vi "Main.vi"() -> ()   [LabVIEW 2022 SP3]
doc: "This Continuous Measurement sample project is based on the Queued Message Handler template.\n\nThe Event Handling Loop generates messages based on user interface actions.\n\nThe Message Handling Loop processes messages generated by the Event Handling Loop, or by other messages. There are also Acquisition and Logging message handling loop subVIs, and a chart updating loop."
uses:
  controls/UI Data.ctl
  controls/UI State.ctl
  support/Message Queue/Enqueue Message (Single).vi
  GlobalVariable/GlobalLongueurOnde.vi
  GlobalVariable/GlobalSet0.vi
  GlobalVariable/GlobalDefaultFolderPath.vi
  <vilib>/Utility/error.llb/Error Cluster From Error Code.vi
  <vilib>/ErrorRing/Error Ring.xnode
  Acquisition/Acquisition.lvlib
  support/User Event - Stop/User Event - Stop.lvlib
  support/Message Queue/Message Queue.lvlib
panel:
  out "Pos Y":dbl
  out "Pos X":dbl
  out "?":dbl[][](graph)
  in  "Mise à 0":bool
  in  "Longueur d'onde du laser":dbl
  in  "Exit":bool
  out "Data":waveform(dbl)[](graph)
  out "Array":variant[](array[variant])
  out "Status":string
  out "Puissance Instantannée":dbl
  in  "Start":bool
  in  "Stop":bool
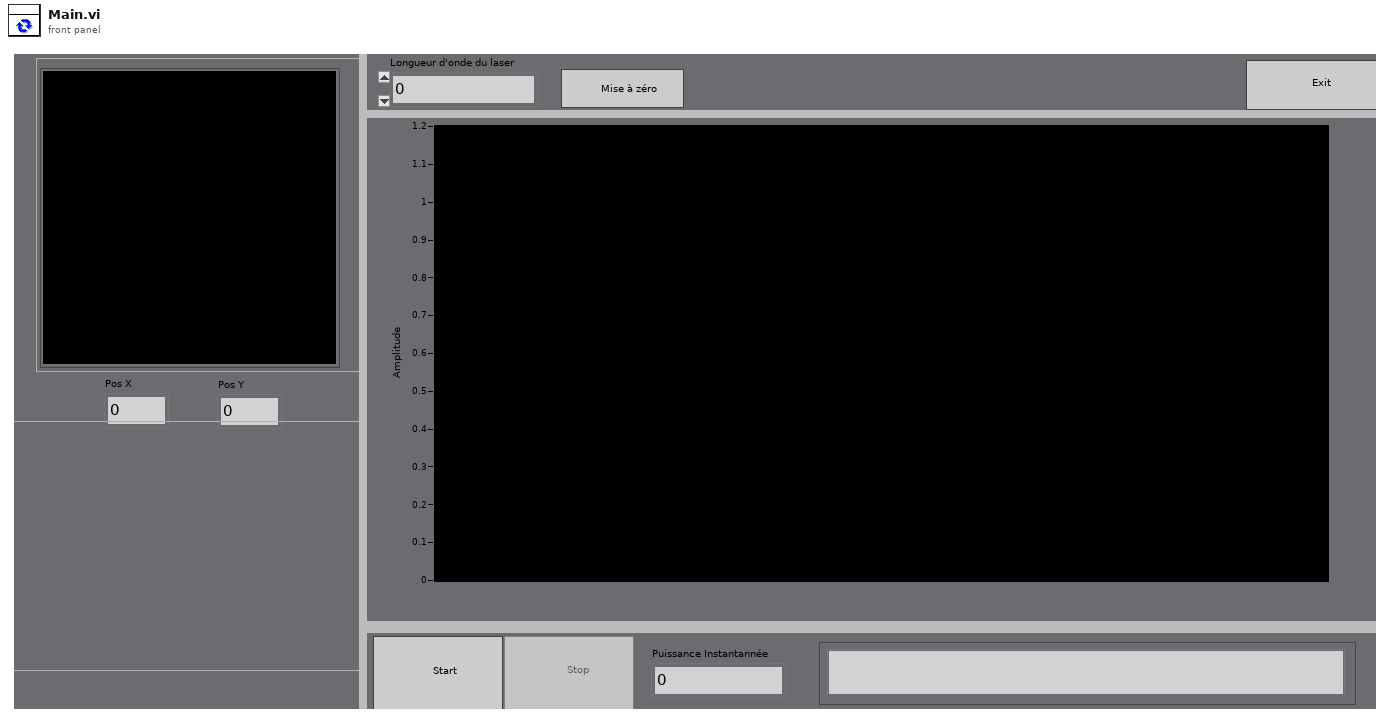
[diagram p1: front panel]
types:
  T1 = typedef "UI State.ctl" = enum16{"Idle", "Acquiring and Logging", "Waiting for Exit", "Waiting for Exit (Acq Stopped)", "Waiting for Exit (Log Stopped)", "Waiting for Stop", "Waiting for Stop (Acq Stopped)", "Waiting for Stop (Log Stopped)"}
  T2 = typedef "UI Data.ctl" = cluster{"Start Ref":refnum<vi>, "Stop Ref":refnum<vi>, "Settings Ref":refnum<vi>, "Exit Ref":refnum<vi>, "Status Ref":refnum<vi>, "Data Ref":refnum<vi>, "Longueur d'onde du laser":refnum<vi>, "Set 0 Ref":refnum<vi>}
  T3 = cluster{"UI":refnum<queue>, "Acquisition":refnum<queue>}
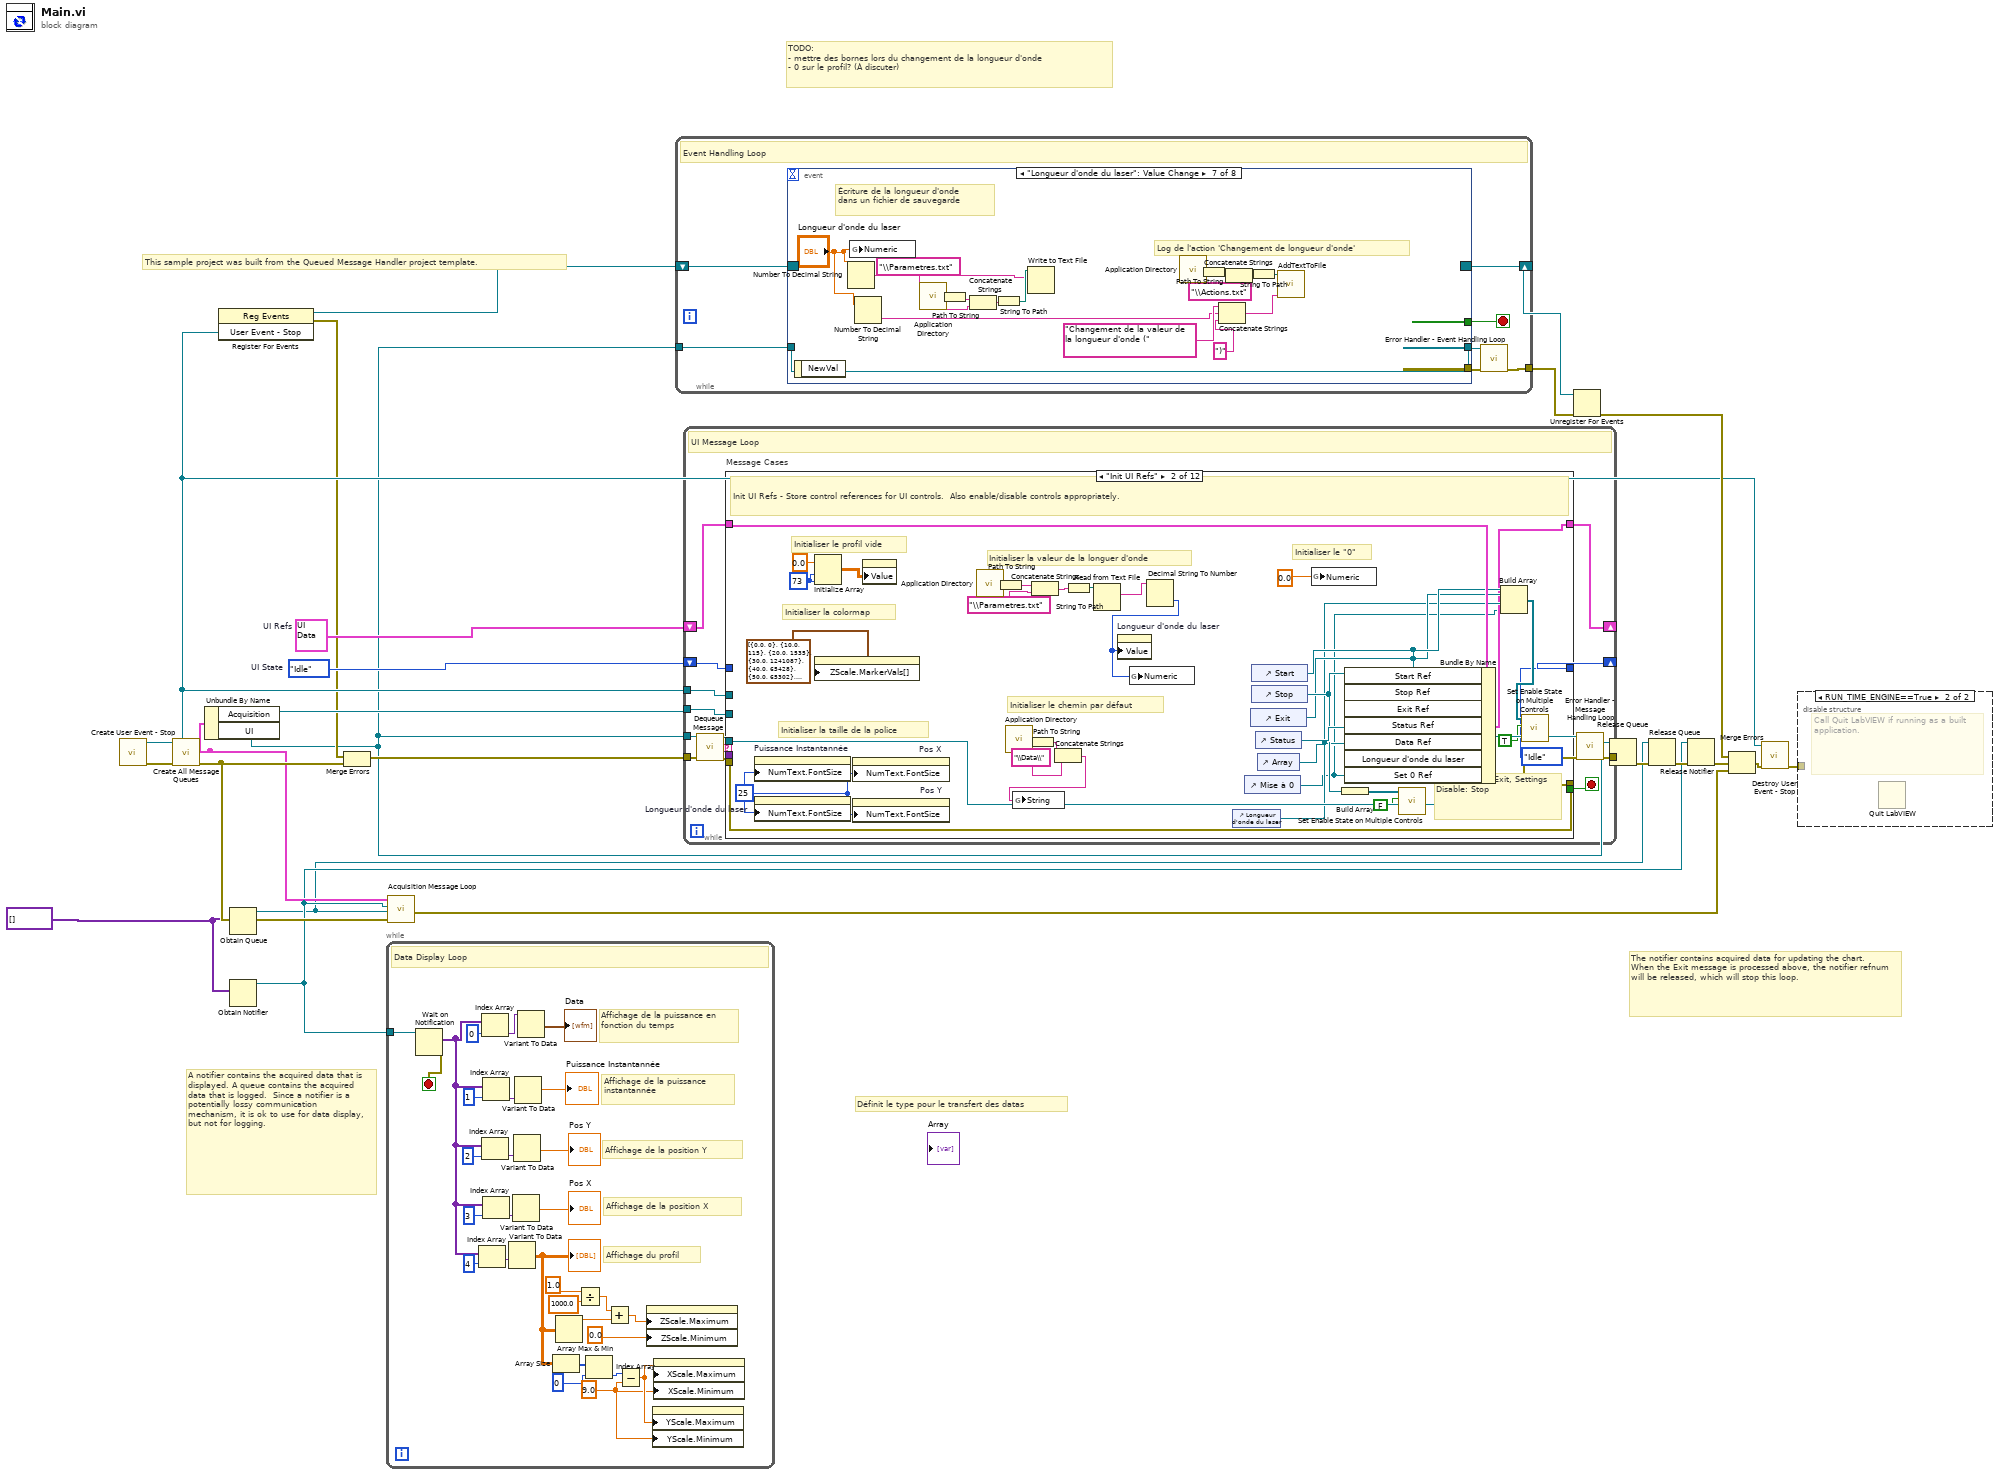
[diagram p0: block diagram]
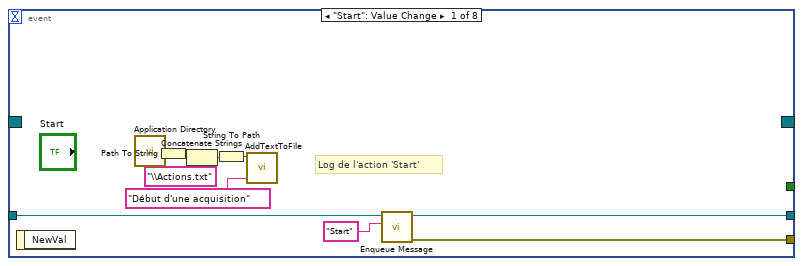
[diagram p3: hidden frame]
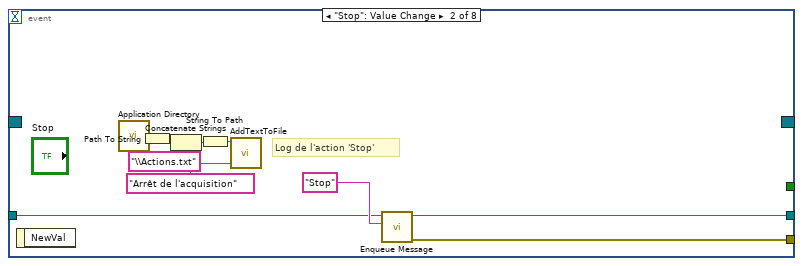
[diagram p4: hidden frame]
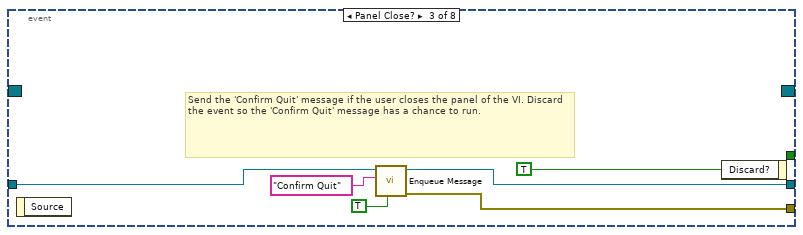
[diagram p5: hidden frame]
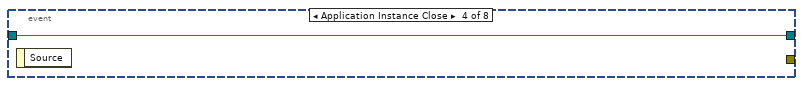
[diagram p6: hidden frame]
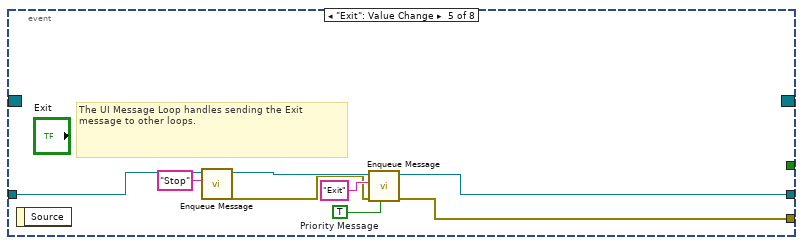
[diagram p7: hidden frame]
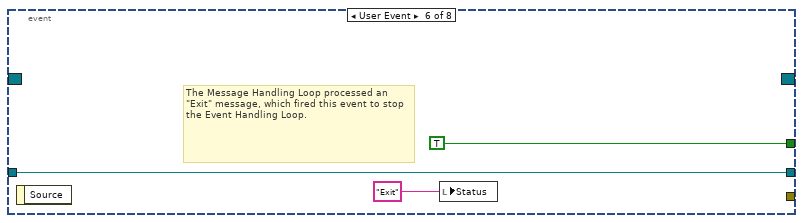
[diagram p8: hidden frame]
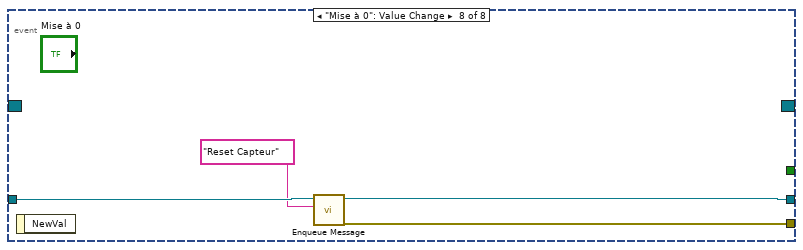
[diagram p9: hidden frame]
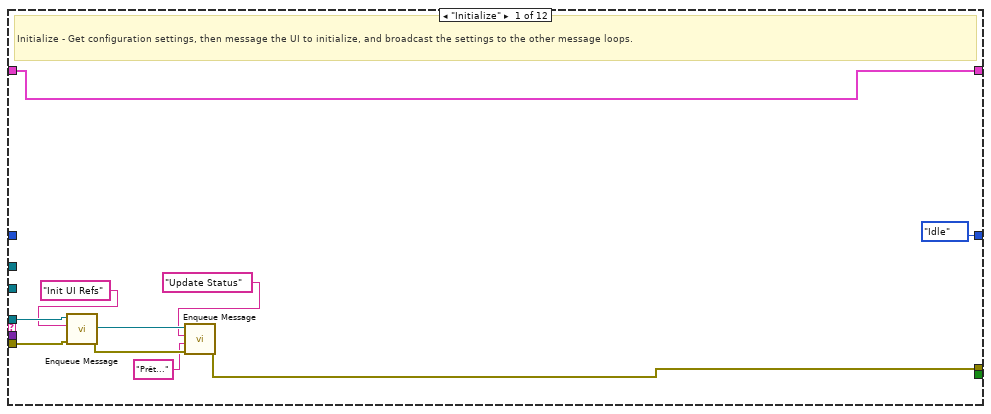
[diagram p10: hidden frame]
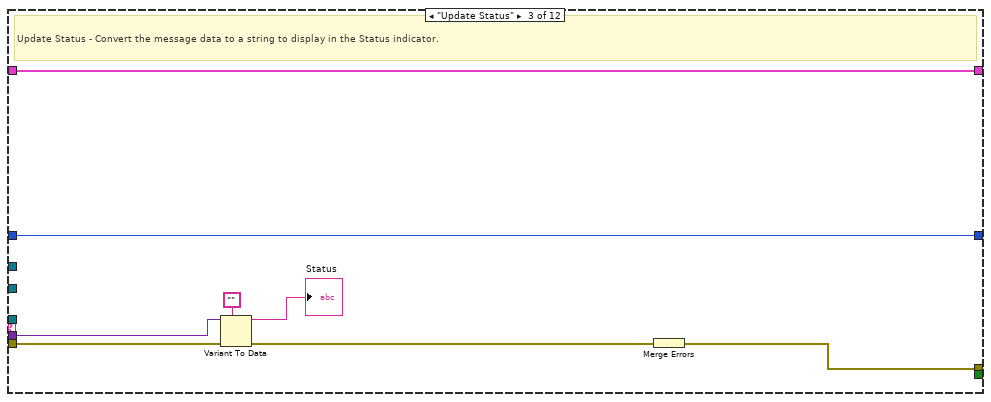
[diagram p11: hidden frame]
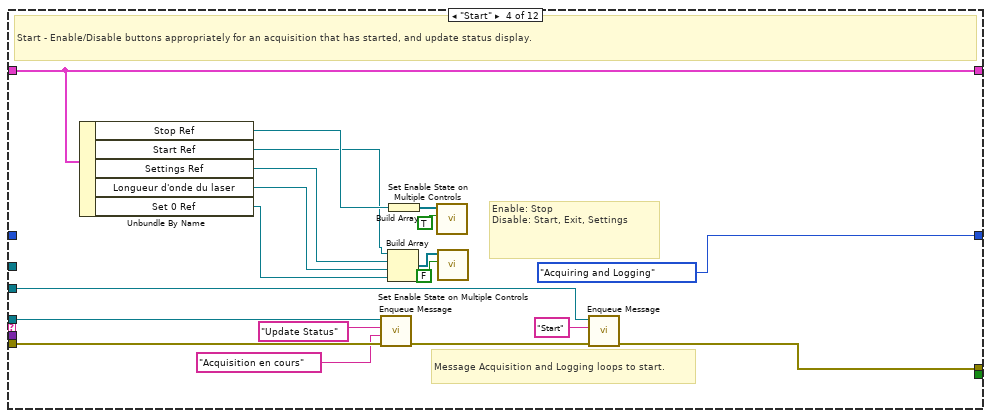
[diagram p12: hidden frame]
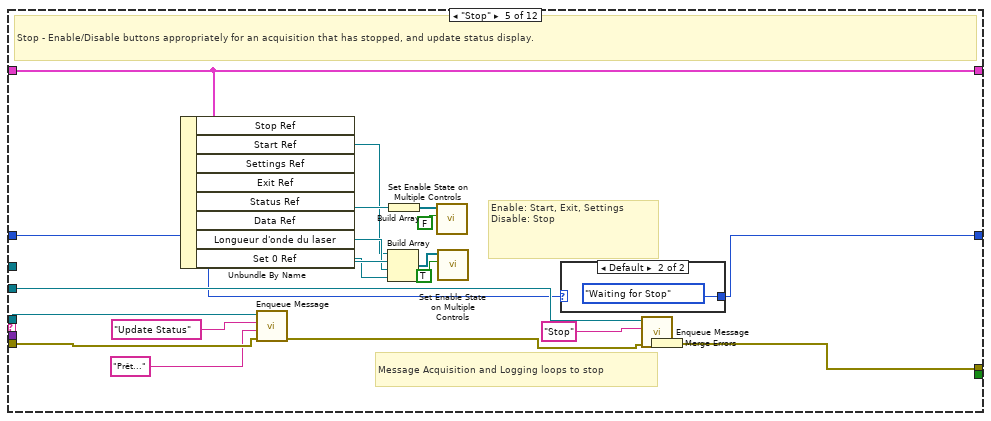
[diagram p13: hidden frame]
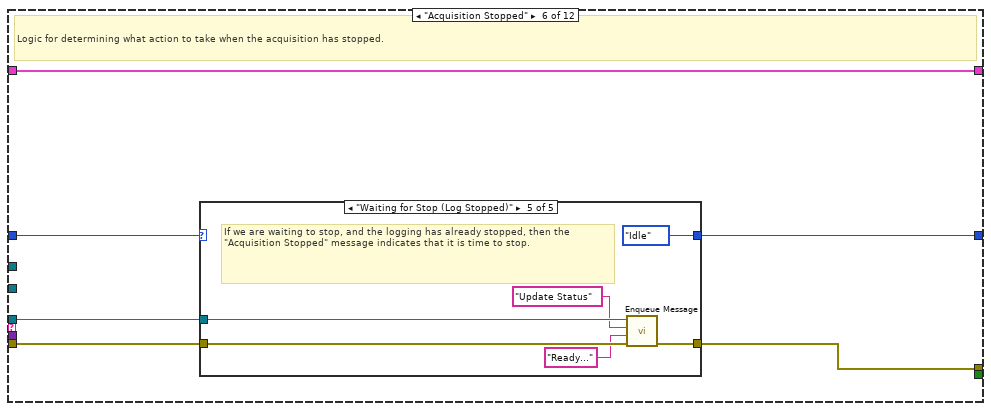
[diagram p15: hidden frame]
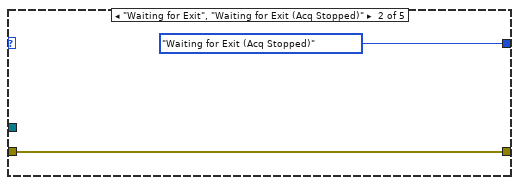
[diagram p17: hidden frame]
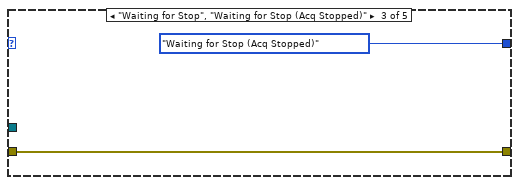
[diagram p18: hidden frame]
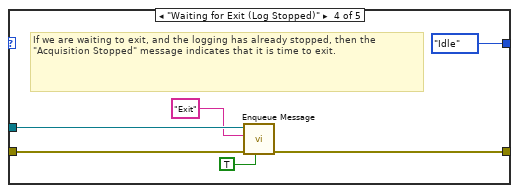
[diagram p19: hidden frame]
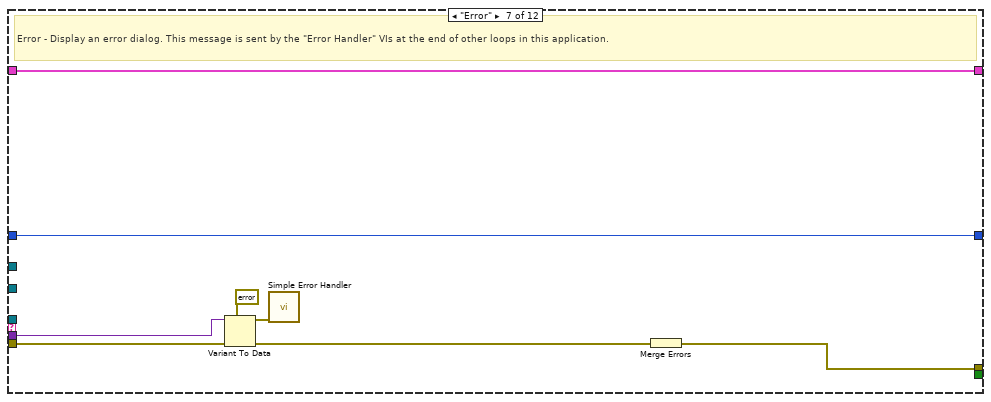
[diagram p20: hidden frame]
diagram:
  w3 = variant[] [] ("appended array")
  w16 = UI_State."Idle"  # UI State
  w18 = T2 {"Start Ref"=refnum, "Stop Ref"=refnum, "Settings Ref"=refnum, "Exit Ref"=refnum, "Status Ref"=refnum, "Data Ref"=refnum, "Longueur d'onde du laser"=refnum, "Set 0 Ref"=refnum}  # UI Refs
  # "TODO: \n- mettre des bornes lors du changement de la longueur d'onde\n- 0 sur le profil? (À discuter)"
  # "Définit le type pour le transfert des datas"
  # "This sample project was built from the Queued Message Handler project template."
  # "A notifier contains the acquired data that is displayed. A queue contains the acquired data that is logged.  Since a notifier is a potentially lossy communication mechanism, it is ok to use for data display, but not for logging."
  # "The notifier contains acquired data for updating the chart. When the Exit message is processed above, the notifier refnum will be released, which will stop this loop."
  n1 = call "Create User Event - Stop.vi"() -> ("error out"=w21:errorcluster, "User Event - Stop"=w9:refnum<user-event>)  [unwired: 10 in]
  n2 = call "Create All Message Queues.vi"("error in (no error)"=w21) -> ("error out"=w20:errorcluster, "Message Queues out"=w4:T3)  [unwired: 9 in]
  n3 = Unbundle By Name(w4) -> ("Acquisition"=w17:refnum<queue>, "UI"=w6:refnum<queue>)
  n4 = register-events(w9) -> (reference out=w10:refnum<event-registration>, error out=w7:errorcluster)  [unwired: 2 in]
  n5 = Obtain Queue(element data type=w3) -> (queue out=w1:refnum<queue>)  [unwired: 4 in, 2 out]
  n6 = Obtain Notifier(notification data type=w3) -> (notifier out=w2:refnum<notifier>)  [unwired: 3 in, 2 out]
  n7 = Merge Errors(w7, w20) -> (w8:errorcluster)
  n8 = while "Data Display Loop" {
    tunnel: w2 -> [w53]
    stop <- w52 stop-if-true
    w46 = 9.0 ("Y Scale.Range:Minimum")
    # "Affichage de la puissance en fonction du temps"
    # "Affichage de la position X"
    # "Affichage de la position Y"
    # "Affichage de la puissance\ninstantannée"
    # "Affichage du profil"
    # "Data Display Loop"
    n9 = Wait on Notification(notifier=w53) -> (notification=w35:variant[], error out=w52:errorcluster)  [unwired: 3 in, 2 out]
    n10 = Index Array(array=w35, index=4) -> (element=w33:variant)
    n11 = Index Array(array=w35, index=0) -> (element=w44:variant)
    n12 = Index Array(array=w35, index=2) -> (element=w39:variant)
    n13 = Index Array(array=w35, index=1) -> (element=w41:variant)
    n14 = Index Array(array=w35, index=3) -> (element=w36:variant)
    n15 = Variant To Data(Variant=w33) -> (data=w32:dbl[][])  [unwired: 2 in, 1 out]
    "?" <- w32
    n16 = Variant To Data(Variant=w36) -> (data=→"Pos X":dbl)  [unwired: 2 in, 1 out]
    n17 = Variant To Data(Variant=w39) -> (data=→"Pos Y":dbl)  [unwired: 2 in, 1 out]
    n18 = Variant To Data(Variant=w41) -> (data=→"Puissance Instantannée":dbl)  [unwired: 2 in, 1 out]
    n19 = Variant To Data(Variant=w44) -> (data=→"Data":waveform(dbl)[])  [unwired: 2 in, 1 out]
    n20 = Array Size(array=w32) -> (size(s)=w50:i32[])
    n21 = Array Max & Min(array=w32) -> (max value=w30:dbl)  [unwired: 3 out]
    n22 = Divide(x=1.0, y=1000.0) -> (x/y=w29:dbl)
    n23 = Index Array(array=w50, index=0) -> (element=w48:i32)
    n24 = Add(x=w29, y=w30) -> (x+y=w31:dbl)
    n25 = Subtract(x=w48, y=w46) -> (x-y=w47:dbl)
    n26 = property class="IntGraph (strict)"("ZScale.Maximum"=w31, "ZScale.Minimum"=0.0 ("Z Scale.Range:Minimum")) -> ()  [unwired: 2 in, 2 out]
    n27 = property class="IntGraph (strict)"("YScale.Maximum"=w47, "YScale.Minimum"=w46) -> ()  [unwired: 2 in, 2 out]
    n28 = property class="IntGraph (strict)"("XScale.Maximum"=w47, "XScale.Minimum"=w46) -> ()  [unwired: 2 in, 2 out]
  }
  n29 = call "Acquisition Message Loop.vi"("error in (no error)"=w20, "queue out"=w1, "Data Notifier"=w2, "Message Queues"=w4) -> ("error out"=w22:errorcluster)  [unwired: 7 in]
  n30 = while {
    tunnel: w6 -> [w59]
    tunnel: [w56] -> w23
    shift-right: [w58] -> w5
    shift-left: w10 -> [w60]
    stop <- w57 stop-if-true
    # "Event Handling Loop"
    n31 = event shown="[6] \"Longueur d'onde du laser\": Value Change" {
      selector: w60 -> [_ _ _ _ _ _ _ _]
      dyn-events: [_ _ _ _ _ _ _ _] -> w58
      timeout: _ -> [_ _ _ _ _ _ _ _]
      tunnel: [_ _ _ _ _ TRUE ("Discard?") _ _] -> w57
      tunnel: w59 -> [w70 w79 w84 w87 w91 w96 w115 w119]
      tunnel: [w68 w78 w82 _ w95 _ _ w117] -> w55
      tunnel: [w67 w77 w83 w87 w92 w96 w115 w118] -> w54
      event "Start": Value Change {
        # "Log de l'action 'Start'"
        n32 = event-data() -> ()  [unwired: 1 in, 1 out]
        n33 = call <vilib>:"Application Directory.vi"() -> ("Application Directory"=w64:path)
        n34 = Path To String(path=w64) -> (string=w65:string)
        n35 = Concatenate Strings(w65, "\\Actions.txt") -> (w66:string)
        n36 = String To Path(string=w66) -> (path=w62:path)
        n37 = call "AddTextToFile.vi"("Ajouter du texte"="Début d'une acquisition", "Fichier"=w62) -> ()  [unwired: 10 in]
        n38 = call-poly "Enqueue Message.vi"("Message"="Start", "Message Queue"=w70) -> ("error out"=w68:errorcluster, "dup Message Queue"=w67:refnum<queue>)  [unwired: 8 in]
      }
      event "Stop": Value Change {
        # "Log de l'action 'Stop'"
        n39 = event-data() -> ()  [unwired: 1 in, 1 out]
        n40 = call <vilib>:"Application Directory.vi"() -> ("Application Directory"=w74:path)
        n41 = Path To String(path=w74) -> (string=w75:string)
        n42 = Concatenate Strings(w75, "\\Actions.txt") -> (w76:string)
        n43 = String To Path(string=w76) -> (path=w72:path)
        n44 = call "AddTextToFile.vi"("Ajouter du texte"="Arrêt de l'acquisition", "Fichier"=w72) -> ()  [unwired: 10 in]
        n45 = call-poly "Enqueue Message.vi"("Message"="Stop", "Message Queue"=w79) -> ("error out"=w78:errorcluster, "dup Message Queue"=w77:refnum<queue>)  [unwired: 8 in]
      }
      event Panel Close? {
        # "Send the 'Confirm Quit' message if the user closes the panel of the VI. Discard the event so the 'Confirm Quit' message has a chance to run."
        n46 = event-data() -> ()  [unwired: 1 in, 1 out]
        n47 = call-poly "Enqueue Message.vi"("Priority Message? (F)"=TRUE, "Message"="Confirm Quit", "Message Queue"=w84) -> ("error out"=w82:errorcluster, "dup Message Queue"=w83:refnum<queue>)  [unwired: 7 in]
        n48 = event-data("Discard?"=TRUE) -> ()  [unwired: 1 in, 1 out]
      }
      event Application Instance Close {
        n49 = event-data() -> ()  [unwired: 1 in, 1 out]
      }
      event "Exit": Value Change {
        w93 = TRUE  # Priority Message
        # "The UI Message Loop handles sending the Exit message to other loops."
        n50 = event-data() -> ()  [unwired: 1 in, 1 out]
        n51 = call-poly "Enqueue Message.vi"("Message"="Stop", "Message Queue"=w91) -> ("error out"=w89:errorcluster, "dup Message Queue"=w90:refnum<queue>)  [unwired: 8 in]
        n52 = call-poly "Enqueue Message.vi"("Priority Message? (F)"=w93, "error in (no error)"=w89, "Message"="Exit", "Message Queue"=w90) -> ("error out"=w95:errorcluster, "dup Message Queue"=w92:refnum<queue>)  [unwired: 6 in]
      }
      event User Event {
        # "The Message Handling Loop processed an \"Exit\" message, which fired this event to stop the Event Handling Loop."
        n53 = event-data() -> ()  [unwired: 1 in, 1 out]
        n54 = local write "Status"("Exit" ("Exit String")) -> ()
      }
      event "Longueur d'onde du laser": Value Change {
        # "Log de l'action 'Changement de longueur d'onde'"
        # "Écriture de la longueur d'onde\ndans un fichier de sauvegarde"
        n55 = event-data() -> ()  [unwired: 1 in, 1 out]
        n56 = Number To Decimal String(number="Longueur d'onde du laser") -> (decimal integer string=w109:string)  [unwired: 1 in]
        n57 = global write "GlobalLongueurOnde.vi" "Numeric"("Longueur d'onde du laser") -> ()
        n58 = Number To Decimal String(number="Longueur d'onde du laser") -> (decimal integer string=w101:string)  [unwired: 1 in]
        n59 = call <vilib>:"Application Directory.vi"() -> ("Application Directory"=w114:path)
        n60 = Path To String(path=w114) -> (string=w113:string)
        n61 = Concatenate Strings(w113, "\\Parametres.txt") -> (w111:string)
        n62 = String To Path(string=w111) -> (path=w110:path)
        n63 = Write to Text File(file (use dialog)=w110, text=w109) -> ()  [unwired: 2 in, 3 out]
        n64 = call <vilib>:"Application Directory.vi"() -> ("Application Directory"=w106:path)
        n65 = Path To String(path=w106) -> (string=w107:string)
        n66 = Concatenate Strings("Changement de la valeur de la longueur d'onde (" ("Ajouter du texte"), w101, ")" ("string")) -> (w99:string)
        n67 = Concatenate Strings(w107, "\\Actions.txt") -> (w108:string)
        n68 = String To Path(string=w108) -> (path=w104:path)
        n69 = call "AddTextToFile.vi"("Ajouter du texte"=w99, "Fichier"=w104) -> ()  [unwired: 10 in]
      }
      event "Mise à 0": Value Change {
        n70 = event-data() -> ()  [unwired: 1 in, 1 out]
        n71 = call-poly "Enqueue Message.vi"("Message"="Reset Capteur", "Message Queue"=w119) -> ("error out"=w117:errorcluster, "dup Message Queue"=w118:refnum<queue>)  [unwired: 8 in]
      }
    }
    n72 = call "Error Handler - Event Handling Loop.vi"("error in (no error)"=w55, "Message Queue"=w54) -> ("dup error in"=w56:errorcluster)  [unwired: 8 in, 1 out]
  }
  n73 = while {
    tunnel: w6 -> [w128]
    tunnel: w9 -> [w133]
    shift-right: [w126] -> _
    shift-left: w18 -> [w127]
    tunnel: w17 -> [w125]
    shift-right: [w120] -> _
    shift-left: w16 -> [w121]
    tunnel: w8 -> [w132]
    tunnel: [w124] -> w24
    stop <- w134 stop-if-true
    # "UI Message Loop"
    n74 = call "Dequeue Message.vi"("error in (no error)"=w132, "Message Queue"=w128) -> ("error out"=w131:errorcluster, "Message Data"=w129:variant, "Message"=w130:string, "dup Message Queue"=w122:refnum<queue>)  [unwired: 6 in]
    n75 = case "Message Cases" shown="\"Init UI Refs\"" w130 {
      selector: w130 -> [_ _ _ _ _ _ _ _ _ _ _ w309]
      tunnel: w122 -> [w139 _ _ w203 w209 w229 _ w262 _ _ _ _]
      tunnel: w131 -> [w138 w176 w183 w202 w207 w230 w251 w261 _ w301 w307 _]
      tunnel: [w136 w176 w184 w192 w224 w227 w254 w260 w295 w300 w306 w308] -> w123
      tunnel: [_ _ _ _ _ _ _ _ TRUE _ _ _] -> w134
      tunnel: w129 -> [_ _ w182 _ _ _ w255 _ w290 _ _ _]
      tunnel: w133 -> [_ _ _ _ _ _ _ _ w296 _ _ _]
      tunnel: w127 -> [w140 w175 w178 w199 w223 w232 w258 w264 w294 w299 w305 w311]
      tunnel: [w140 w162 w178 w199 w223 w232 w258 w264 w294 w299 w305 w311] -> w126
      tunnel: w125 -> [_ _ _ w191 w215 _ _ _ w287 _ _ _]
      tunnel: w121 -> [_ _ w177 _ w212 w231 w253 w263 _ w298 w304 w310]
      tunnel: [UI_State."Idle" ("UI State") UI_State."Idle" ("UI State") w177 UI_State."Acquiring and Logging" ("UI State") w213 w228 w253 w259 UI_State."Idle" ("UI State") w298 w304 w310] -> w120
      frame "Initialize" {
        # "Initialize - Get configuration settings, then message the UI to initialize, and broadcast the settings to the other message loops."
        n76 = call-poly "Enqueue Message.vi"("error in (no error)"=w138, "Message"="Init UI Refs", "Message Queue"=w139) -> ("error out"=w144:errorcluster, "dup Message Queue"=w143:refnum<queue>)  [unwired: 7 in]
        n77 = call-poly "Enqueue Message.vi"("error in (no error)"=w144, "Message Data"="Prêt..." ("Ready..."), "Message"="Update Status", "Message Queue"=w143) -> ("error out"=w136:errorcluster)  [unwired: 6 in, 1 out]
      }
      frame "Init UI Refs" {
        w149 = 73 ("dimension size")
        w164 = 25
        # "Initialiser le \"0\""
        # "Initialiser le profil vide"
        # "Initialiser la valeur de la longuer d'onde"
        # "Initialiser le chemin par défaut"
        # "Initialiser la colormap"
        # "Initialiser la taille de la police"
        # "Enable: Start, Exit, Settings\nDisable: Stop"
        # "Init UI Refs - Store control references for UI controls.  Also enable/disable controls appropriately."
        n78 = property on="Puissance Instantannée" class="DigNum (strict)"("NumText.FontSize"=w164) -> ()  [unwired: 2 in, 2 out]
        n79 = property on="Longueur d'onde du laser" class="DigNum (strict)"("NumText.FontSize"=w164) -> ()  [unwired: 2 in, 2 out]
        n80 = property class="IntGraph (strict)"("ZScale.MarkerVals[]"=cluster{dbl, u32}[] [{0.0, 0}, {10.0, 115}, {20.0, 1535}, {30.0, 1241087}, {40.0, 65428}, {50.0, 65302}, {60.0, 15925010}, {70.0, 16756736}, {80.0, 16739858}, {90.0, 16712704}, {100.0, 10420224}] ("Z Scale.Marker Values[]")) -> ()  [unwired: 2 in, 2 out]
        n81 = Initialize Array(0.0 ("element"), w149, w149) -> (w148:dbl[][])
        n82 = property on="Pos X" class="DigNum (strict)"("NumText.FontSize"=w164) -> ()  [unwired: 2 in, 2 out]
        n83 = property on="Pos Y" class="DigNum (strict)"("NumText.FontSize"=w164) -> ()  [unwired: 2 in, 2 out]
        n84 = property class="IntGraph (strict)"("Value"=w148) -> ()  [unwired: 2 in, 2 out]
        n85 = call <vilib>:"Application Directory.vi"() -> ("Application Directory"=w158:path)
        n86 = Path To String(path=w158) -> (string=w157:string)
        n87 = call <vilib>:"Application Directory.vi"() -> ("Application Directory"=w161:path)
        n88 = Path To String(path=w161) -> (string=w160:string)
        n89 = Concatenate Strings(w157, "\\Parametres.txt") -> (w156:string)
        n90 = Concatenate Strings(w160, "\\Data\\") -> (w146:string)
        n91 = global write "GlobalDefaultFolderPath.vi" "String"(w146) -> ()
        n92 = String To Path(string=w156) -> (path=w155:path)
        n93 = Read from Text File(file (use dialog)=w155) -> (text=w153:string)  [unwired: 3 in, 3 out]
        n94 = Decimal String To Number(string=w153) -> (number=w152:i32)  [unwired: 2 in, 1 out]
        n95 = property on="Longueur d'onde du laser" class="DigNum (strict)"("Value"=w152) -> ()  [unwired: 2 in, 2 out]
        n96 = global write "GlobalLongueurOnde.vi" "Numeric"(w152) -> ()
        n97 = control-ref of="Longueur d'onde du laser"() -> (w165:refnum<vi>)
        n98 = control-ref of="Mise à 0"() -> (w147:refnum<vi>)
        n99 = control-ref of="Exit"() -> (w167:refnum<vi>)
        n100 = control-ref of="Start"() -> (w168:refnum<vi>)
        n101 = control-ref of="Stop"() -> (w169:refnum<vi>)
        n102 = control-ref of="Status"() -> (w174:refnum<vi>)
        n103 = control-ref of="Array"() -> (w151:refnum<vi>)
        n104 = global write "GlobalSet0.vi" "Numeric"(0.0) -> ()
        n105 = Build Array(w169) -> (w171:refnum<vi>[])
        n106 = Bundle By Name(cluster=w175, "Start Ref"=w168, "Stop Ref"=w169, "Exit Ref"=w167, "Status Ref"=w174, "Data Ref"=w151, "Longueur d'onde du laser"=w165, "Set 0 Ref"=w147) -> (w162:T2)
        n107 = call "Set Enable State on Multiple Controls.vi"("Enable?"=FALSE, "Controls"=w171) -> ()  [unwired: 10 in]
        n108 = Build Array(w168, w167, w165, w147) -> (w172:refnum<vi>[])
        n109 = call "Set Enable State on Multiple Controls.vi"("Enable?"=TRUE, "Controls"=w172) -> ()  [unwired: 10 in]
      }
      frame "Update Status" {
        # "Update Status - Convert the message data to a string to display in the Status indicator."
        n110 = Variant To Data(error in=w183, type="", Variant=w182) -> (data=→"Status":string, error out=w180:errorcluster)
        n111 = Merge Errors(w180) -> (w184:errorcluster)
      }
      frame "Start" {
        # "Message Acquisition and Logging loops to start."
        # "Enable: Stop\nDisable: Start, Exit, Settings"
        # "Start - Enable/Disable buttons appropriately for an acquisition that has started, and update status display."
        n112 = Unbundle By Name(w199) -> ("Stop Ref"=w194:refnum<vi>, "Start Ref"=w187:refnum<vi>, "Settings Ref"=w193:refnum<vi>, "Longueur d'onde du laser"=w188:refnum<vi>, "Set 0 Ref"=w185:refnum<vi>)
        n113 = call-poly "Enqueue Message.vi"("error in (no error)"=w202, "Message Data"="Acquisition en cours" ("Acquiring and Logging..."), "Message"="Update Status", "Message Queue"=w203) -> ("error out"=w186:errorcluster)  [unwired: 6 in, 1 out]
        n114 = Build Array(w187, w193, w188, w185) -> (w197:refnum<vi>[])
        n115 = Build Array(w194) -> (w196:refnum<vi>[])
        n116 = call "Set Enable State on Multiple Controls.vi"("Enable?"=TRUE, "Controls"=w196) -> ()  [unwired: 10 in]
        n117 = call "Set Enable State on Multiple Controls.vi"("Enable?"=FALSE, "Controls"=w197) -> ()  [unwired: 10 in]
        n118 = call-poly "Enqueue Message.vi"("error in (no error)"=w186, "Message"="Start", "Message Queue"=w191) -> ("error out"=w192:errorcluster)  [unwired: 7 in, 1 out]
      }
      frame "Stop" {
        # "Message Acquisition and Logging loops to stop"
        # "Enable: Start, Exit, Settings\nDisable: Stop"
        # "Stop - Enable/Disable buttons appropriately for an acquisition that has stopped, and update status display."
        n119 = Unbundle By Name(w223) -> ("Stop Ref"=w218:refnum<vi>, "Start Ref"=w210:refnum<vi>, "Settings Ref"=w217:refnum<vi>, "Longueur d'onde du laser"=w211:refnum<vi>, "Set 0 Ref"=w204:refnum<vi>)  [unwired: 3 out]
        n120 = call-poly "Enqueue Message.vi"("error in (no error)"=w207, "Message Data"="Prêt..." ("Acquiring and Logging..."), "Message"="Update Status", "Message Queue"=w209) -> ("error out"=w205:errorcluster)  [unwired: 6 in, 1 out]
        n121 = Build Array(w210, w217, w211, w204) -> (w221:refnum<vi>[])
        n122 = Build Array(w218) -> (w220:refnum<vi>[])
        n123 = call "Set Enable State on Multiple Controls.vi"("Enable?"=FALSE, "Controls"=w220) -> ()  [unwired: 10 in]
        n124 = call "Set Enable State on Multiple Controls.vi"("Enable?"=TRUE, "Controls"=w221) -> ()  [unwired: 10 in]
        n125 = case shown="Default" w212 {
          selector: w212 -> [w225 _]
          tunnel: [w225 UI_State."Waiting for Stop" ("UI State")] -> w213
          frame "Waiting for Exit" {
          }
          frame Default {
          }
        }
        n126 = call-poly "Enqueue Message.vi"("error in (no error)"=w205, "Message"="Stop", "Message Queue"=w215) -> ("error out"=w216:errorcluster)  [unwired: 7 in, 1 out]
        n127 = Merge Errors(w216) -> (w224:errorcluster)
      }
      frame "Acquisition Stopped" {
        # "Logic for determining what action to take when the acquisition has stopped."
        n128 = case shown="\"Waiting for Stop (Log Stopped)\"" w231 {
          selector: w231 -> [w234 _ _ _ _]
          tunnel: w230 -> [w233 w236 w238 w244 w250]
          tunnel: w229 -> [_ _ _ w242 w247]
          tunnel: [w234 UI_State."Waiting for Exit (Acq Stopped)" ("UI State") UI_State."Waiting for Stop (Acq Stopped)" ("UI State") UI_State."Idle" ("UI State") UI_State."Idle" ("UI State")] -> w228
          tunnel: [w233 w236 w238 w243 w248] -> w227
          frame Default {
          }
          frame "Waiting for Exit", "Waiting for Exit (Acq Stopped)" {
          }
          frame "Waiting for Stop", "Waiting for Stop (Acq Stopped)" {
          }
          frame "Waiting for Exit (Log Stopped)" {
            # "If we are waiting to exit, and the logging has already stopped, then the \"Acquisition Stopped\" message indicates that it is time to exit."
            n129 = call-poly "Enqueue Message.vi"("Priority Message? (F)"=TRUE, "error in (no error)"=w244, "Message"="Exit", "Message Queue"=w242) -> ("error out"=w243:errorcluster)  [unwired: 6 in, 1 out]
          }
          frame "Waiting for Stop (Log Stopped)" {
            # "If we are waiting to stop, and the logging has already stopped, then the \"Acquisition Stopped\" message indicates that it is time to stop."
            n130 = call-poly "Enqueue Message.vi"("error in (no error)"=w250, "Message Data"="Ready..." ("Ready..."), "Message"="Update Status", "Message Queue"=w247) -> ("error out"=w248:errorcluster)  [unwired: 6 in, 1 out]
          }
        }
      }
      frame "Error" {
        # "Error - Display an error dialog. This message is sent by the \"Error Handler\" VIs at the end of other loops in this application."
        n131 = Variant To Data(error in=w251, type=errorcluster {"status"=FALSE, "code"=0, "source"=""} ("error constant"), Variant=w255) -> (data=w252:errorcluster, error out=w256:errorcluster)
        n132 = call <vilib>:"Simple Error Handler.vi"("error in (no error)"=w252) -> ()  [unwired: 4 in, 5 out]
        n133 = Merge Errors(w256) -> (w254:errorcluster)
      }
      frame "Confirm Quit" {
        # "Confirm Quit - Message that can confirm whether or not the user wants to exit the application."
        n134 = case shown="\"Acquiring and Logging\"" w263 {
          tunnel: w262 -> [w270 w274]
          tunnel: w261 -> [w269 w273]
          tunnel: [w268 w272] -> w260
          tunnel: [UI_State."Idle" ("UI State") w271] -> w259
          frame Default {
            # "If 'Confirm Quit' comes in while the system is idle, there is no need for a confirmation message."
            n135 = call-poly "Enqueue Message.vi"("Priority Message? (F)"=TRUE, "error in (no error)"=w269, "Message"="Exit", "Message Queue"=w270) -> ("error out"=w268:errorcluster)  [unwired: 6 in, 1 out]
          }
          frame "Acquiring and Logging" {
            n136 = Two Button Dialog(message="Are you sure you want to quit while the acquisition is running?" ("Confirm Quit Message"), 1:"No" ("No"), 2:"Yes" ("Yes")) -> (T button?=w275:bool)
            n137 = case shown="True" w275 {
              tunnel: w274 -> [_ w284]
              tunnel: w273 -> [w280 w285]
              tunnel: [w280 w283] -> w272
              tunnel: [UI_State."Acquiring and Logging" ("UI State") UI_State."Waiting for Exit" ("UI State")] -> w271
              frame False {
                # "User did not want to quit."
              }
              frame True {
                n138 = call-poly "Enqueue Message.vi"("error in (no error)"=w285, "Message"="Stop", "Message Queue"=w284) -> ("error out"=w283:errorcluster)  [unwired: 7 in, 1 out]
              }
            }
          }
        }
      }
      frame "Exit" {
        # "Popup an error dialog if 'Exit' was called as a result of an error."
        # "Stop the VI"
        # "Exit - Send Exit messages to the Acquisition and Logging loops, and fire the user event to stop the Event Handling Loop."
        n139 = Variant To Data(type=errorcluster {"status"=FALSE, "code"=0, "source"=""} ("error constant"), Variant=w290) -> (data=w289:errorcluster)  [unwired: 1 in, 1 out]
        n140 = call <vilib>:"Simple Error Handler.vi"("error in (no error)"=w289) -> ()  [unwired: 4 in, 5 out]
        n141 = call-poly "Enqueue Message.vi"("Priority Message? (F)"=FALSE, "Message"="Exit", "Message Queue"=w287) -> ("error out"=w286:errorcluster)  [unwired: 7 in, 1 out]
        n142 = call "Fire User Event - Stop.vi"("error in (no error)"=w286, "User Event - Stop"=w296) -> ("error out"=w295:errorcluster)  [unwired: 9 in]
      }
      frame "---Copy This Frame---" {
        # "Duplicate this frame when creating new messages.  Change this comment in the duplicated frame to describe this message."
        n143 = Merge Errors(w301) -> (w300:errorcluster)
      }
      frame "Reset Capteur" {
        # "Duplicate this frame when creating new messages.  Change this comment in the duplicated frame to describe this message."
        n144 = global read "GlobalLongueurOnde.vi" "Numeric"() -> (w302:dbl)
        n145 = call "SetTo0.vi"("Longueur d'onde"=w302) -> ("Tension 0"=w303:dbl)  [unwired: 10 in]
        n146 = global write "GlobalSet0.vi" "Numeric"(w303) -> ()
        n147 = Merge Errors(w307) -> (w306:errorcluster)
      }
      frame Default {
        # "'Default' case only runs if there is a message that isn't defined in any of the other cases.  Output a programming error."
        n148 = xnode "Error Ring"("parameter 0"=w309) -> ("error out"=w308:errorcluster)
      }
    }
    n149 = call "Error Handler - Message Handling Loop.vi"("error in (no error)"=w123, "Message Queue"=w122) -> ("dup error in"=w124:errorcluster)  [unwired: 8 in, 1 out]
  }
  n150 = Unregister For Events(event registration refnum=w5, error in=w23) -> (error out=w19:errorcluster)
  n151 = Release Queue(queue=w6, error in (no error)=w24) -> (error out=w13:errorcluster)  [unwired: 1 in, 2 out]
  n152 = Release Queue(queue=w1, error in (no error)=w13) -> (error out=w12:errorcluster)  [unwired: 1 in, 2 out]
  n153 = Release Notifier(notifier=w2, error in (no error)=w12) -> (error out=w11:errorcluster)  [unwired: 1 in, 2 out]
  n154 = Merge Errors(w19, w11, w22) -> (w15:errorcluster)
  n155 = call "Destroy User Event - Stop.vi"("error in (no error)"=w15, "User Event - Stop"=w9) -> ("error out"=w14:errorcluster)  [unwired: 9 in]
  n156 = disable-structure shown="RUN_TIME_ENGINE==True" {
    disable-tunnel: w14 -> [_ _]
    frame condition #0 (active) {
    }
    frame condition #1 {
      # "Call Quit LabVIEW if running as a built application."
      n157 = Quit LabVIEW() -> ()  [unwired: 1 in]
    }
  }
